vi "writeBGBatch.vi"(8 "ROI Parameters":T1, 9 "Drop Time (ms)":dbl, 10 "Scan name":string, 11 "file (use dialog)":path) -> ()   [LabVIEW 2016]
uses:
  Controls/ScanParameters/ROI_set.ctl
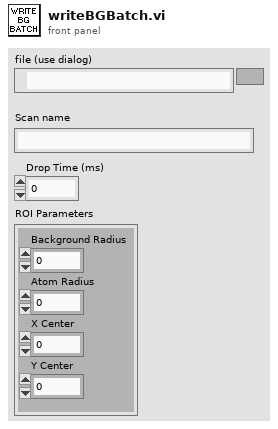
[diagram p1: front panel]
types:
  T1 = typedef "ROI_set.ctl" = cluster{"Background Radius":dbl, "Atom Radius":dbl, "X Center":dbl, "Y Center":dbl}
  T2 = enum16{"open", "replace", "create", "open or create", "replace or create", "replace or create with confirmation"}
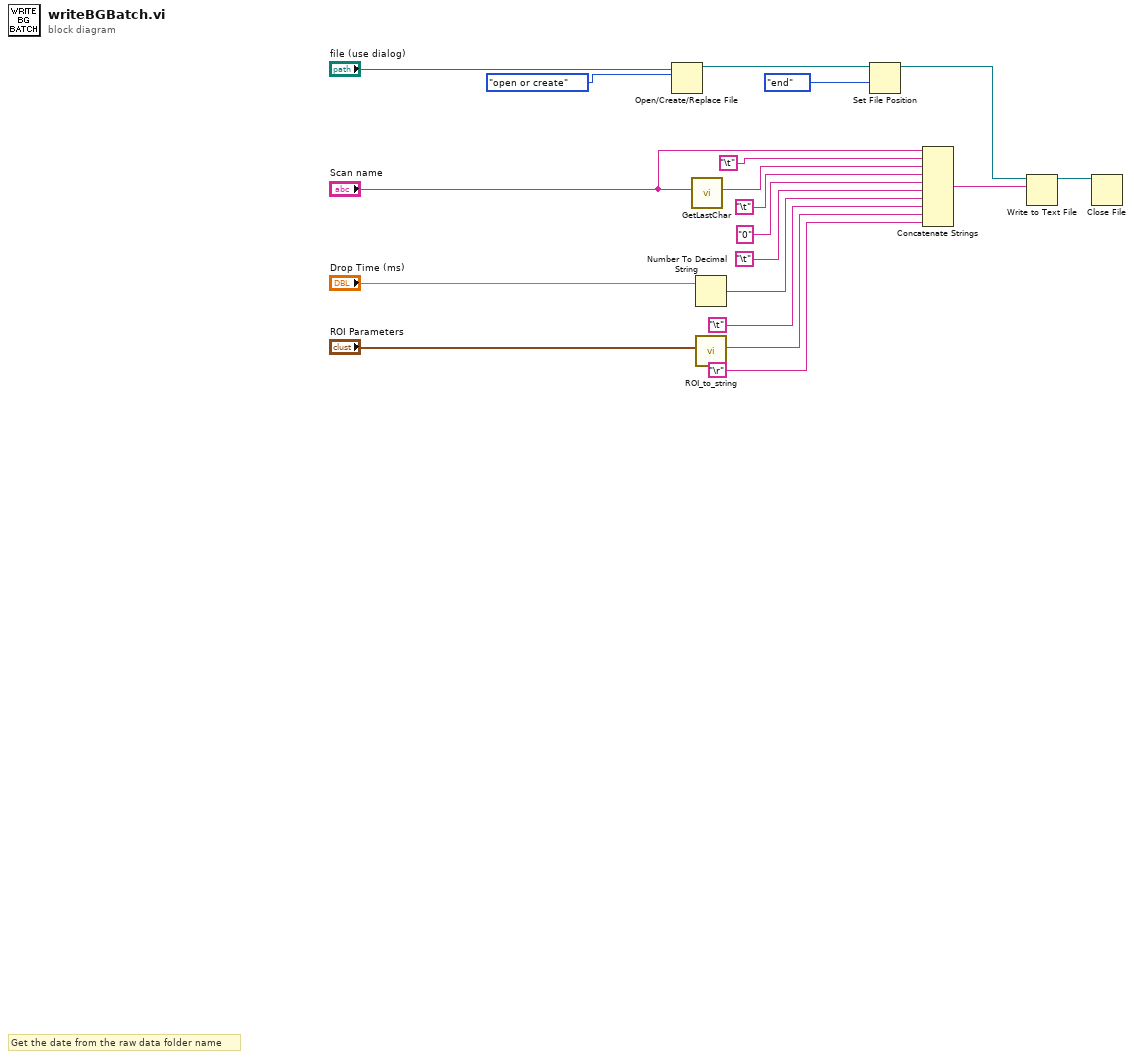
[diagram p0: block diagram]
diagram:
  # "Get the date from the raw data folder name"
  n1 = Open/Create/Replace File(file path (use dialog)="file (use dialog)", operation (0:open)=T2."open or create") -> (refnum out=w5:refnum<file>)  [unwired: 4 in, 2 out]
  n2 = call "GetLastChar.vi"("String"="Scan name") -> ("String 2"=w14:string)  [unwired: 10 in]
  n3 = Number To Decimal String(number="Drop Time (ms)") -> (decimal integer string=w8:string)  [unwired: 1 in]
  n4 = call "ROI_to_string.vi"("ROI Parameters"="ROI Parameters") -> ("String"=w10:string)  [unwired: 10 in]
  n5 = Set File Position(refnum=w5, from (0:start)=enum16{"start", "end", "current"}."end") -> (refnum out=w3:refnum<file>)  [unwired: 2 in, 1 out]
  n6 = Concatenate Strings("Scan name", "\t", w14, "\t", "0" ("string"), "\t", w8, "\t", w10, "\r") -> (w17:string)
  n7 = Write to Text File(file (use dialog)=w3, text=w17) -> (refnum out=w2:refnum<file>)  [unwired: 2 in, 2 out]
  n8 = Close File(refnum=w2) -> ()  [unwired: 1 in, 2 out]
